vi "proyecto HM MF.vi"() -> ()   [LabVIEW 2021]
uses:
  <vilib>/LabVIEW Interface for Arduino/Type Defs/Pin Mode.ctl
  <vilib>/LabVIEW Interface for Arduino/LabVIEW Interface for Arduino.lvlib
panel:
  in  "On":bool
  in  "Paro":bool
  out "Bomba 3":bool
  out "Bomba 2":bool
  out "Bomba1":bool
  in  "Selector 3":enum16{"Sin-alcohol", "Con-alcohol"}(ring)=enum."Con-alcohol"
  # "Cubaneitor"
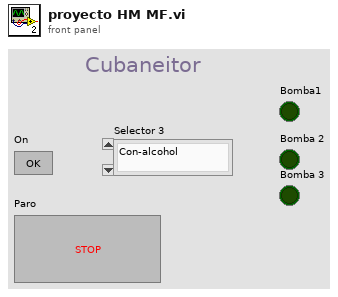
[diagram p1: front panel]
types:
  T1 = typedef "LabVIEW Interface for Arduino.lvlib/Pin Mode.ctl" = enum8{"Input", "Output"}
  T2 = typedef "LabVIEW Interface for Arduino.lvlib/Arduino Resource.ctl" = cluster{"VISA resource":refnum<visa-resource-name>, "Board Type":T3, "Connection Type":enum8{"USB / Serial"}, "Bytes Per Packet (15)":u8}
  T3 = typedef "LabVIEW Interface for Arduino.lvlib/Board Type.ctl" = enum16{"Uno", "Dimuelanove w/Atmega 328", "Mega 2560"}
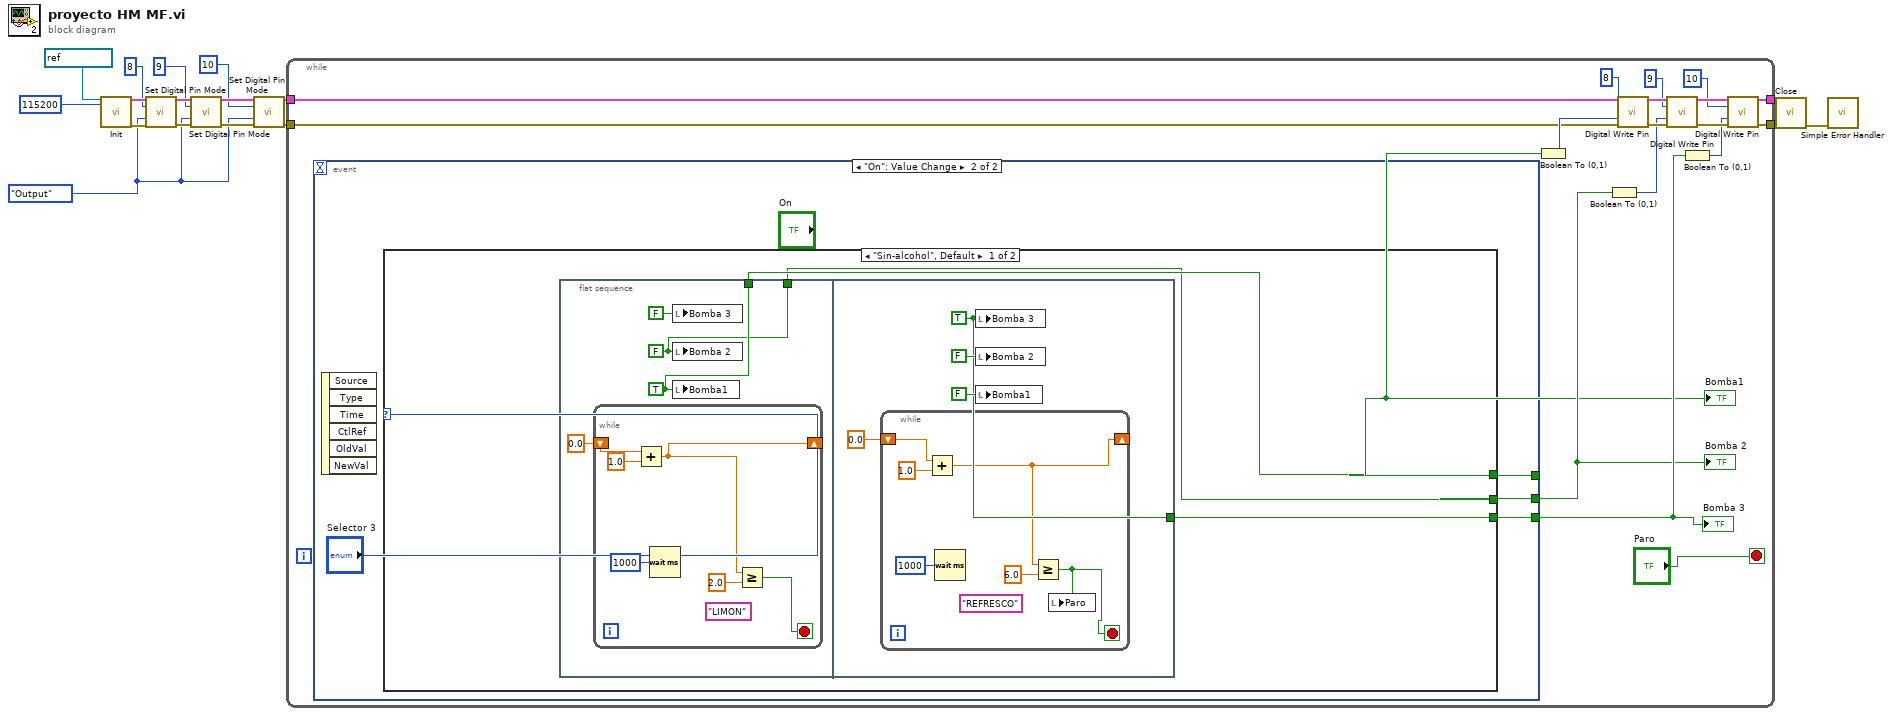
[diagram p0: block diagram]
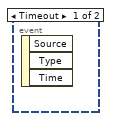
[diagram p2: hidden frame]
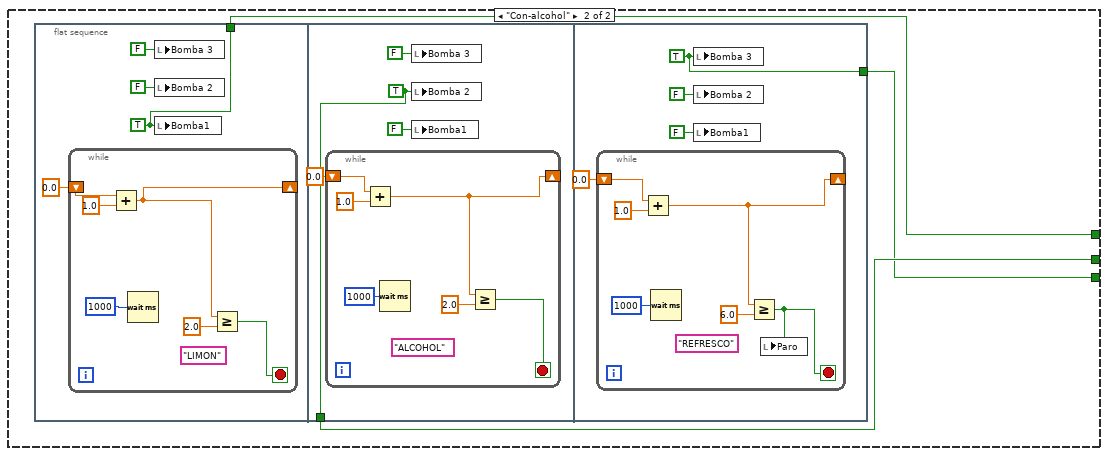
[diagram p3: hidden frame]
diagram:
  w9 = Pin_Mode."Output" ("Pin Mode (Input)")
  n1 = call <vilib>:"Init.vi"("VISA resource"=refnum<visa-resource-name> "COM10", "Baud Rate (115200)"=u32 115200) -> ("Arduino Resource"=w10:T2, "error out"=w15:errorcluster)  [unwired: 16 in]
  n2 = call <vilib>:"Set Digital Pin Mode.vi"("Arduino Resource"=w10, "Digital I/O Pin"=u8 8, "Pin Mode (Input)"=w9, "error in"=w15) -> ("Arduino Resource"=w11:T2, "error out"=w14:errorcluster)  [unwired: 10 in]
  n3 = call <vilib>:"Set Digital Pin Mode.vi"("Arduino Resource"=w11, "Digital I/O Pin"=u8 9, "Pin Mode (Input)"=w9, "error in"=w14) -> ("Arduino Resource"=w12:T2, "error out"=w13:errorcluster)  [unwired: 10 in]
  n4 = call <vilib>:"Set Digital Pin Mode.vi"("Arduino Resource"=w12, "Digital I/O Pin"=u8 10, "Pin Mode (Input)"=w9, "error in"=w13) -> ("Arduino Resource"=w5:T2, "error out"=w4:errorcluster)  [unwired: 10 in]
  n5 = while {
    tunnel: w5 -> [w25]
    tunnel: w4 -> [w24]
    tunnel: [w23] -> w2
    tunnel: [w22] -> w1
    stop <- "Paro" stop-if-true
    n6 = event shown="[1] \"On\": Value Change" {
      selector: _ -> [_ _]
      dyn-events: _ -> [_ _]
      timeout: _ -> [_ _]
      tunnel: [_ w38] -> w18
      tunnel: [_ w37] -> w20
      tunnel: [_ w36] -> w21
      event Timeout {
        n7 = event-data() -> ()  [unwired: 1 in, 3 out]
      }
      event "On": Value Change {
        n8 = event-data() -> ()  [unwired: 1 in, 6 out]
        n9 = case shown="\"Sin-alcohol\", Default" "Selector 3" {
          tunnel: [w42 w65] -> w38
          tunnel: [w40 w64] -> w37
          tunnel: [w41 w63] -> w36
          frame "Sin-alcohol", Default {
            n10 = flat-sequence {
              tunnel: [w44] -> w42
              tunnel: [w43] -> w40
              tunnel: [w53] -> w41
              frame #0 {
                w43 = FALSE ("Bomba 2")
                w44 = TRUE ("Bomba1")
                n11 = while {
                  shift-right: [w50] -> _
                  shift-left: 0.0 -> [w52]
                  stop <- w48 stop-if-true
                  (unwired) "LIMON"
                  n12 = Add(x=w52, y=1.0) -> (x+y=w50:dbl)
                  n13 = Wait (ms)(milliseconds to wait=u32 1000) -> ()  [unwired: 1 out]
                  n14 = Greater Or Equal?(x=w50, y=2.0) -> (x >= y?=w48:bool)
                }
                n15 = local write "Bomba 3"(FALSE ("Bomba 3")) -> ()
                n16 = local write "Bomba 2"(w43) -> ()
                n17 = local write "Bomba1"(w44) -> ()
              }
              frame #1 {
                w53 = TRUE ("Bomba 3")
                n18 = while {
                  shift-right: [w60] -> _
                  shift-left: 0.0 -> [w58]
                  stop <- w57 stop-if-true
                  (unwired) "REFRESCO"
                  n19 = Add(x=w58, y=1.0) -> (x+y=w60:dbl)
                  n20 = Wait (ms)(milliseconds to wait=u32 1000) -> ()  [unwired: 1 out]
                  n21 = Greater Or Equal?(x=w60, y=6.0) -> (x >= y?=w57:bool)
                  n22 = local write "Paro"(w57) -> ()
                }
                n23 = local write "Bomba 3"(w53) -> ()
                n24 = local write "Bomba 2"(FALSE ("Bomba 2")) -> ()
                n25 = local write "Bomba1"(FALSE ("Bomba1")) -> ()
              }
            }
          }
          frame "Con-alcohol" {
            n26 = flat-sequence {
              tunnel: [w67] -> w65
              tunnel: [w77] -> w64
              tunnel: [w87] -> w63
              frame #0 {
                w67 = TRUE ("Bomba1")
                n27 = while {
                  shift-right: [w73] -> _
                  shift-left: 0.0 -> [w75]
                  stop <- w71 stop-if-true
                  (unwired) "LIMON"
                  n28 = Add(x=w75, y=1.0) -> (x+y=w73:dbl)
                  n29 = Wait (ms)(milliseconds to wait=u32 1000) -> ()  [unwired: 1 out]
                  n30 = Greater Or Equal?(x=w73, y=2.0) -> (x >= y?=w71:bool)
                }
                n31 = local write "Bomba 3"(FALSE ("Bomba 3")) -> ()
                n32 = local write "Bomba 2"(FALSE ("Bomba 2")) -> ()
                n33 = local write "Bomba1"(w67) -> ()
              }
              frame #1 {
                w77 = TRUE ("Bomba 2")
                n34 = while {
                  shift-right: [w83] -> _
                  shift-left: 0.0 -> [w80]
                  stop <- w82 stop-if-true
                  (unwired) "ALCOHOL"
                  n35 = Add(x=w80, y=1.0) -> (x+y=w83:dbl)
                  n36 = Wait (ms)(milliseconds to wait=u32 1000) -> ()  [unwired: 1 out]
                  n37 = Greater Or Equal?(x=w83, y=2.0) -> (x >= y?=w82:bool)
                }
                n38 = local write "Bomba 3"(FALSE ("Bomba 3")) -> ()
                n39 = local write "Bomba 2"(w77) -> ()
                n40 = local write "Bomba1"(FALSE ("Bomba1")) -> ()
              }
              frame #2 {
                w87 = TRUE ("Bomba 3")
                n41 = while {
                  shift-right: [w93] -> _
                  shift-left: 0.0 -> [w91]
                  stop <- w90 stop-if-true
                  (unwired) "REFRESCO"
                  n42 = Add(x=w91, y=1.0) -> (x+y=w93:dbl)
                  n43 = Wait (ms)(milliseconds to wait=u32 1000) -> ()  [unwired: 1 out]
                  n44 = Greater Or Equal?(x=w93, y=6.0) -> (x >= y?=w90:bool)
                  n45 = local write "Paro"(w90) -> ()
                }
                n46 = local write "Bomba 3"(w87) -> ()
                n47 = local write "Bomba 2"(FALSE ("Bomba 2")) -> ()
                n48 = local write "Bomba1"(FALSE ("Bomba1")) -> ()
              }
            }
          }
        }
      }
    }
    "Bomba1" <- w18
    "Bomba 2" <- w20
    "Bomba 3" <- w21
    n49 = Boolean To (0,1)(Boolean=w18) -> (0, 1=w31:i16)
    n50 = Boolean To (0,1)(Boolean=w20) -> (0, 1=w30:i16)
    n51 = call <vilib>:"Digital Write Pin.vi"("Arduino Resource"=w25, "Digital I/O Pin (0)"=u8 8, "Value (0)"=w31, "error in"=w24) -> ("Arduino Resource"=w32:T2, "error out"=w33:errorcluster)  [unwired: 10 in]
    n52 = call <vilib>:"Digital Write Pin.vi"("Arduino Resource"=w32, "Digital I/O Pin (0)"=u8 9, "Value (0)"=w30, "error in"=w33) -> ("Arduino Resource"=w35:T2, "error out"=w34:errorcluster)  [unwired: 10 in]
    n53 = Boolean To (0,1)(Boolean=w21) -> (0, 1=w29:i16)
    n54 = call <vilib>:"Digital Write Pin.vi"("Arduino Resource"=w35, "Digital I/O Pin (0)"=u8 10, "Value (0)"=w29, "error in"=w34) -> ("Arduino Resource"=w22:T2, "error out"=w23:errorcluster)  [unwired: 10 in]
  }
  n55 = call <vilib>:"Close.vi"("Arduino Resource"=w1, "error in"=w2) -> ("error out"=w3:errorcluster)  [unwired: 13 in]
  n56 = call <vilib>:"Simple Error Handler.vi"("error in (no error)"=w3) -> ()  [unwired: 4 in, 5 out]
